vi "Create file name.vi"(8 "error in (no error)":errorcluster, 11 "Tomo in":refnum<class "Tomo.lvclass">) -> (0 "error out":errorcluster, 2 "filename":string, 3 "Tomo out":refnum<class "Tomo.lvclass">)   [LabVIEW 2012, in "Tomo.lvclass"]
uses:
  Tomo.lvclass
  Tomo.lvclass/Tomo.ctl
  <vilib>/Distrio/Murmex/Murmex/Murmex.lvclass
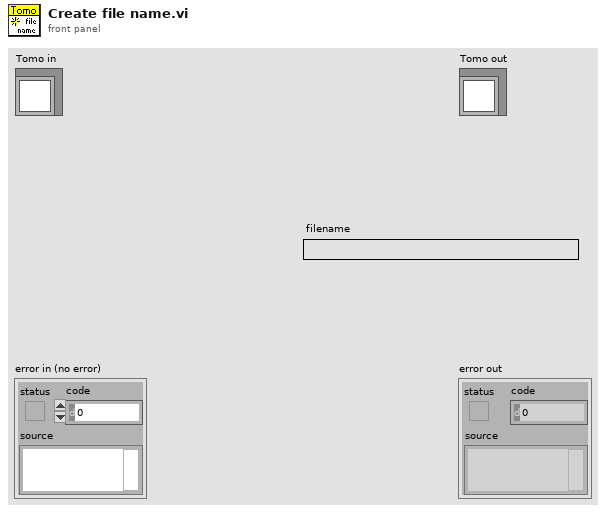
[diagram p1: front panel]
types:
  T1 = typedef "Tomo.lvclass/Current activity.ctl" = enum16{"Idle", "Inter-stack motion", "Pre-tomo calculation", "Stack acquisition", "Stack preparation", "Pre-tomo stack acq", "Pre-tomo inter-stack"}
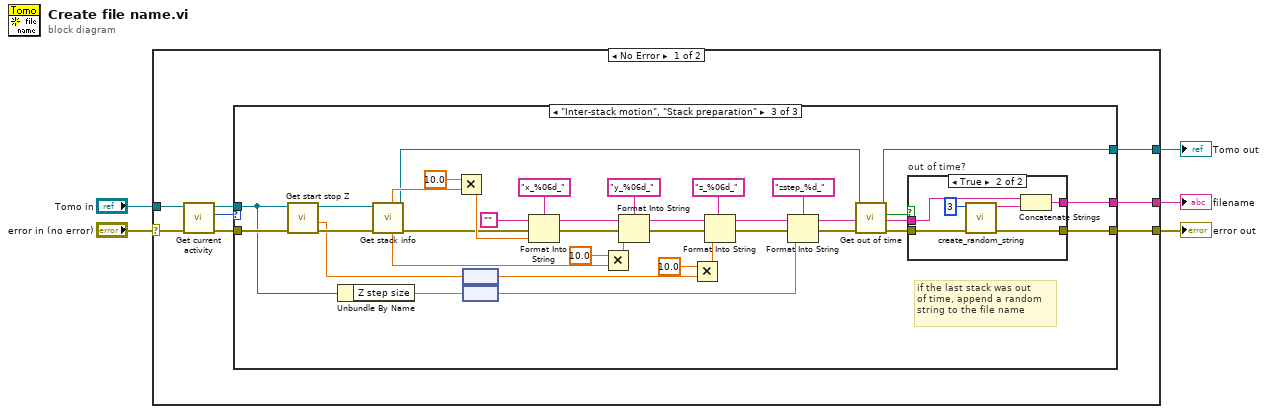
[diagram p0: block diagram]
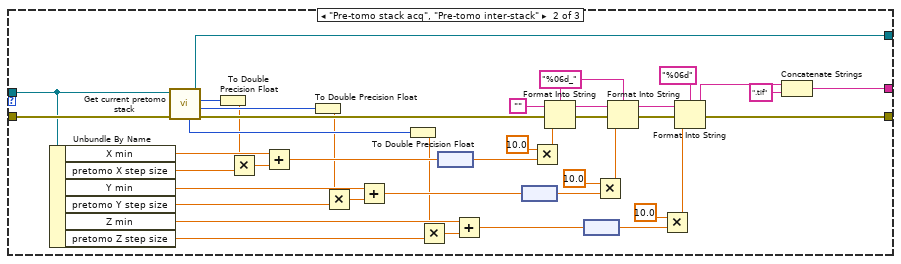
[diagram p3: hidden frame]
diagram:
  n1 = case shown="No Error" "error in (no error)" {
    selector: "error in (no error)" -> [w10 w103]
    tunnel: [w13 w103] -> w4
    tunnel: [w11 w102] -> w2
    tunnel: "Tomo in" -> [w8 w102]
    tunnel: [w12 _] -> w1
    frame No Error {
      n2 = call-dynamic "Get current activity.vi"("error in (no error)"=w10, "Tomo in"=w8) -> ("error out"=w9:errorcluster, "Current activity"=w6:T1, "Tomo out"=w7:refnum<class "Tomo.lvclass">)  [unwired: 7 in]
      n3 = case shown="\"Inter-stack motion\", \"Stack preparation\"" w6 {
        tunnel: [w14 w31 w70] -> w13
        tunnel: [_ w27 w68] -> w12
        tunnel: [w15 w52 w65] -> w11
        tunnel: w9 -> [w14 w57 w59]
        tunnel: w7 -> [w15 w51 w58]
        frame "Idle", Default {
        }
        frame "Pre-tomo stack acq", "Pre-tomo inter-stack" {
          w26 = "%06d_" ("format string")
          n4 = Unbundle By Name(w51) -> ("X min"=w45:dbl[unit], "pretomo X step size"=w50:dbl[unit], "Y min"=w39:dbl[unit], "pretomo Y step size"=w40:dbl[unit], "Z min"=w35:dbl[unit], "pretomo Z step size"=w36:dbl[unit])
          n5 = call-dynamic "Get current pretomo stack.vi"("error in (no error)"=w57, "Tomo in"=w51) -> ("error out"=w55:errorcluster, "y loop number"=w48:i32, "x loop number"=w49:i32, "Tomo out"=w52:refnum<class "Tomo.lvclass">, "z step number"=w47:i32)  [unwired: 5 in]
          n6 = To Double Precision Float(number=w49) -> (double precision float=w44:dbl)
          n7 = Multiply(x=w44, y=w50) -> (x*y=w46:dbl[unit])
          n8 = Add(x=w45, y=w46) -> (x+y=w43:dbl[unit])
          n9 = To Double Precision Float(number=w48) -> (double precision float=w38:dbl)
          n10 = Multiply(x=w38, y=w40) -> (x*y=w42:dbl[unit])
          n11 = Add(x=w39, y=w42) -> (x+y=w37:dbl[unit])
          n12 = To Double Precision Float(number=w47) -> (double precision float=w34:dbl)
          n13 = Multiply(x=w34, y=w36) -> (x*y=w41:dbl[unit])
          n14 = node(w43) -> (w23:dbl)
          n15 = Add(x=w35, y=w41) -> (x+y=w33:dbl[unit])
          n16 = node(w37) -> (w21:dbl)
          n17 = Multiply(x=10.0, y=w23) -> (x*y=w22:dbl)
          n18 = Format Into String(format string=w26, initial string="", error in=w55, w22) -> (resulting string=w53:string, error out=w54:errorcluster)
          n19 = node(w33) -> (w18:dbl)
          n20 = Multiply(x=10.0, y=w21) -> (x*y=w19:dbl)
          n21 = Format Into String(format string=w26, initial string=w53, error in=w54, w19) -> (resulting string=w30:string, error out=w32:errorcluster)
          n22 = Multiply(x=10.0, y=w18) -> (x*y=w17:dbl)
          n23 = Format Into String(format string="%06d", initial string=w30, error in=w32, w17) -> (resulting string=w28:string, error out=w31:errorcluster)
          n24 = Concatenate Strings(w28, ".tif" ("string")) -> (w27:string)
        }
        frame "Inter-stack motion", "Stack preparation" {
          # "if the last stack was out\nof time, append a random\nstring to the file name"
          n25 = call-dynamic "Get start stop Z.vi"("error in (no error)"=w59, "Tomo in"=w58) -> ("error out"=w63:errorcluster, "Z start"=w61:dbl[unit], "Tomo out"=w62:refnum<class "Tomo.lvclass">)  [unwired: 4 in, 3 out]
          n26 = Unbundle By Name(w58) -> ("Z step size"=w77:dbl[unit])
          n27 = call-dynamic "Get stack info.vi"("error in (no error)"=w63, "Tomo in"=w62) -> ("error out"=w90:errorcluster, "Tomo out"=w66:refnum<class "Tomo.lvclass">, "Y position"=w80:dbl, "X position"=w92:dbl)  [unwired: 3 in, 3 out]
          n28 = Multiply(x=10.0, y=w92) -> (x*y=w93:dbl)
          n29 = node(w61) -> (w60:dbl)
          n30 = node(w77) -> (w76:dbl)
          n31 = Format Into String(format string="x_%06d_", initial string="", error in=w90, w93) -> (resulting string=w83:string, error out=w89:errorcluster)
          n32 = Multiply(x=10.0, y=w80) -> (x*y=w79:dbl)
          n33 = Format Into String(format string="y_%06d_", initial string=w83, error in=w89, w79) -> (resulting string=w82:string, error out=w88:errorcluster)
          n34 = Multiply(x=10.0, y=w60) -> (x*y=w78:dbl)
          n35 = Format Into String(format string="z_%06d_", initial string=w82, error in=w88, w78) -> (resulting string=w81:string, error out=w87:errorcluster)
          n36 = Format Into String(format string="zstep_%d_", initial string=w81, error in=w87, w76) -> (resulting string=w69:string, error out=w71:errorcluster)
          n37 = call-dynamic "Get out of time.vi"("error in (no error)"=w71, "Tomo in"=w66) -> ("error out"=w67:errorcluster, "out of time?"=w64:bool, "Tomo out"=w65:refnum<class "Tomo.lvclass">)  [unwired: 7 in]
          n38 = case "out of time?" shown="True" w64 {
            tunnel: w67 -> [w94 w101]
            tunnel: [w94 w100] -> w70
            tunnel: w69 -> [w95 w98]
            tunnel: [w95 w97] -> w68
            frame False {
            }
            frame True {
              n39 = call <vilib>:"create_random_string.vi"("error in (no error)"=w101, "length"=3) -> ("error out"=w100:errorcluster, "random string"=w96:string)  [unwired: 8 in]
              n40 = Concatenate Strings(w98, w96) -> (w97:string)
            }
          }
        }
      }
    }
    frame Error {
    }
  }
  "error out" <- w4
  "Tomo out" <- w2
  "filename" <- w1
